vi "Check_Type_of_Merging(101)-1.vi"(1 "[IN] Subtracks":T1(array[cluster])) -> (0 "[OUT] # of Additional Costs":i32)   [LabVIEW 2013]
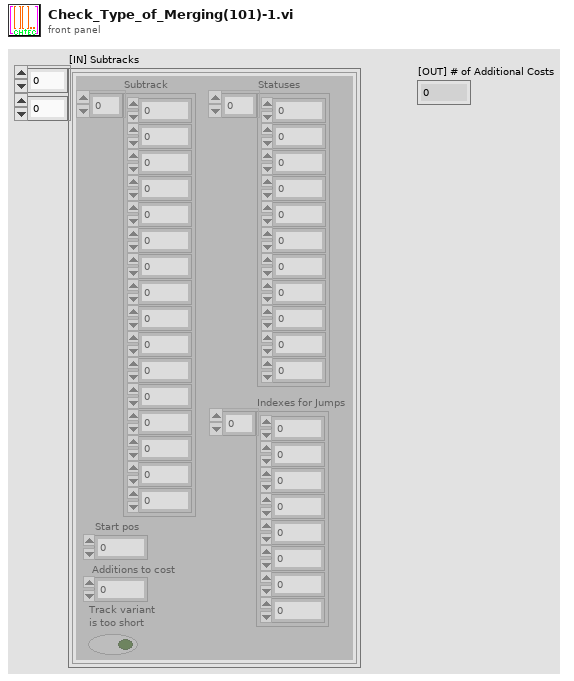
[diagram p1: front panel]
types:
  T1 = cluster{"Subtrack":dbl[], "Statuses":i16[], "Start pos":i32, "Additions to cost":i32, "Track variant \nis too short":bool, "Indexes for Jumps":i32[]}[][]
  T2 = cluster{"Subtrack":dbl[], "Statuses":i16[], "Start pos":i32, "Additions to cost":i32, "Track variant \nis too short":bool, "Indexes for Jumps":i32[]}[]
  T3 = cluster{"Subtrack":dbl[], "Statuses":i16[], "Start pos":i32, "Additions to cost":i32, "Track variant \nis too short":bool, "Indexes for Jumps":i32[]}
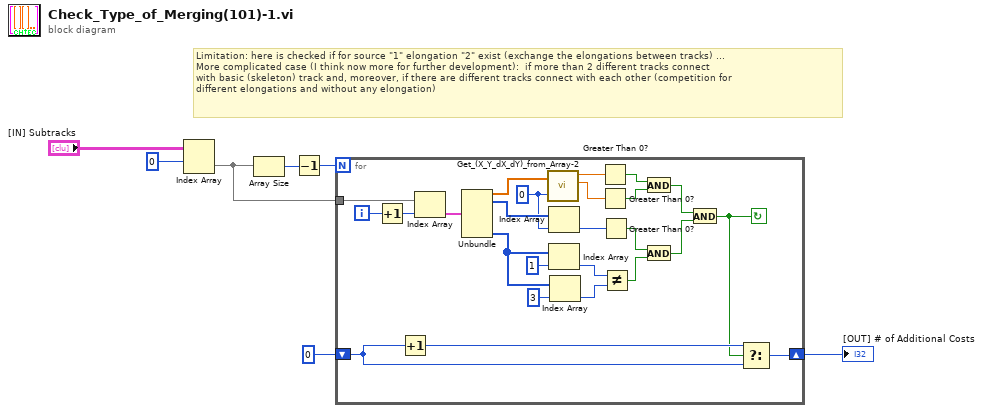
[diagram p0: block diagram]
diagram:
  # "Limitation: here is checked if for source \"1\" elongation \"2\" exist (exchange the elongations between tracks) ... \nMore complicated case (I think now more for further development):  if more than 2 different tracks connect \nwith basic (skeleton) track and, moreover, if there are different tracks connect with each other (competition for \ndifferent elongations and without any elongation)"
  n1 = Index Array(array="[IN] Subtracks", index (row)=0) -> (element=w5:T2)  [unwired: 1 in]
  n2 = Array Size(array=w5) -> (size(s)=w3:i32)
  n3 = Decrement(x=w3) -> (x-1=w2:i32)
  n4 = for {
    N: w2 -> [_]
    tunnel: w5 -> [w32]
    shift-right: [w9] -> w1
    shift-left: 0 ("disabled index (col)") -> [w10]
    i -> [w24]
    stop <- w8 continue-if-true
    w28 = 0
    n5 = Increment(x=w24) -> (x+1=w23:i32)
    n6 = Increment(x=w10) -> (x+1=w11:i32)
    n7 = Index Array(array=w32, index=w23) -> (element=w31:T3)
    n8 = Unbundle(w31) -> ("Subtrack"=w30:dbl[], "Statuses"=w29:i16[], "Indexes for Jumps"=w20:i32[])  [unwired: 3 out]
    n9 = call "Get_(X_Y_dX_dY)_from_Array-2.vi"("(X,Y,dX,dY)"=w30, "Index of Displacement"=w28) -> ("X"=w27:dbl, "Y"=w26:dbl)  [unwired: 2 out]
    n10 = Index Array(array=w29, index=w28) -> (element=w25:i16)
    n11 = Index Array(array=w20, index=1) -> (element=w19:i32)
    n12 = Index Array(array=w20, index=3) -> (element=w18:i32)
    n13 = Greater Than 0?(x=w27) -> (x > 0?=w17:bool)
    n14 = Greater Than 0?(x=w26) -> (x > 0?=w16:bool)
    n15 = Greater Than 0?(x=w25) -> (x > 0?=w15:bool)
    n16 = Not Equal?(x=w19, y=w18) -> (x != y?=w14:bool)
    n17 = And(x=w17, y=w16) -> (x .and. y?=w13:bool)
    n18 = And(x=w15, y=w14) -> (x .and. y?=w12:bool)
    n19 = And(x=w13, y=w12) -> (x .and. y?=w8:bool)
    n20 = Select(t=w11, s=w8, f=w10) -> (s? t:f=w9:i32)
  }
  "[OUT] # of Additional Costs" <- w1
